vi "IntegralTerm.vi"(0 "Error":dbl format="%#_13g", 1 "Arm kI":dbl format="%#_13g", 4 "Reset I?":bool) -> (7 "I":dbl format="%#_13g")   [LabVIEW 2014]
panel:
  in  "I_Cap":dbl format="%#_13g"
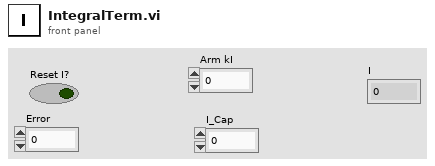
[diagram p1: front panel]
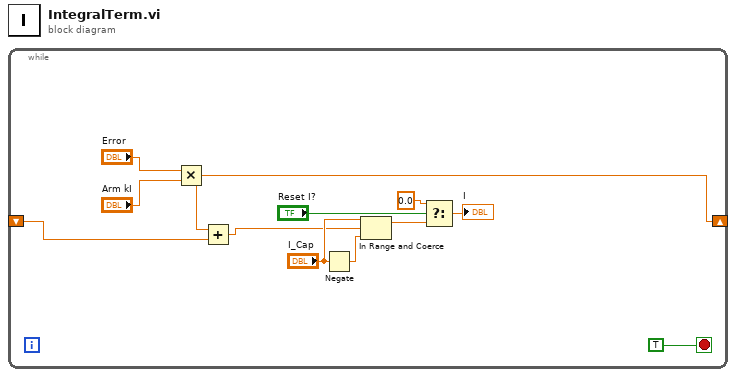
[diagram p0: block diagram]
diagram:
  n1 = while {
    shift-right: [w8] -> _
    shift-left: _ -> [w7]
    stop <- TRUE stop-if-true
    n2 = Multiply(x="Error", y="Arm kI") -> (x*y=w8:dbl)
    n3 = Add(x=w8, y=w7) -> (x+y=w4:dbl)
    n4 = Negate(x="I_Cap") -> (-x=w11:dbl)
    n5 = In Range and Coerce(upper limit="I_Cap", x=w4, lower limit=w11) -> (coerced(x)=w3:dbl)  [unwired: 1 out]
    n6 = Select(t=0.0, s="Reset I?", f=w3) -> (s? t:f=→"I":dbl)
  }
